vi "Read Connection Information.vi"(8 "error in (no error)":errorcluster, 11 "TwinCAT ADS in":refnum<class "TwinCAT ADS.lvclass">) -> (0 "error out":errorcluster, 1 "Connection Information":T1, 3 "TwinCAT ADS out":refnum<class "TwinCAT ADS.lvclass">)   [LabVIEW 2018, in "TwinCAT ADS.lvclass"]
uses:
  TwinCAT ADS.lvclass
  Controls/Connection Information.ctl
  Controls/Address.ctl
  Controls/Connection Protocol.ctl
  Controls/Router State.ctl
  Controls/Connection State.ctl
  TwinCAT ADS.lvclass/TwinCAT ADS.ctl
  TwinCAT.Ads
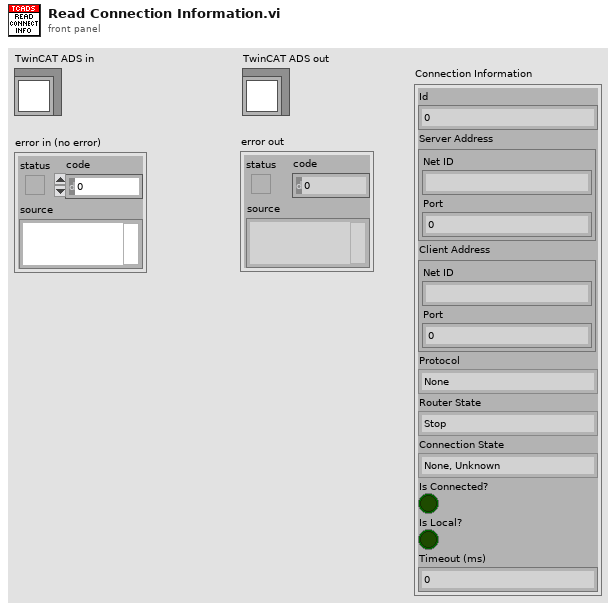
[diagram p1: front panel]
types:
  T1 = typedef "TwinCAT ADS.lvclass/Connection Information.ctl" = cluster{"Id":i32, "Server Address":T2, "Client Address":cluster{"Net ID":string, "Port":i32}, "Protocol":T3, "Router State":T4, "Connection State":T5, "Is Connected?":bool, "Is Local?":bool, "Timeout (ms)":i32}
  T2 = typedef "TwinCAT ADS.lvclass/Address.ctl" = cluster{"Net ID":string, "Port":i32}
  T3 = typedef "TwinCAT ADS.lvclass/Connection Protocol.ctl" = enum16{"None", "Router", "TCP/IP", "All"}
  T4 = typedef "TwinCAT ADS.lvclass/Router State.ctl" = enum16{"Stop", "Start", "Removed", "Unknown"}
  T5 = typedef "TwinCAT ADS.lvclass/Connection State.ctl" = enum16{"None, Unknown", "Disconnected", "Connected", "Lost"}
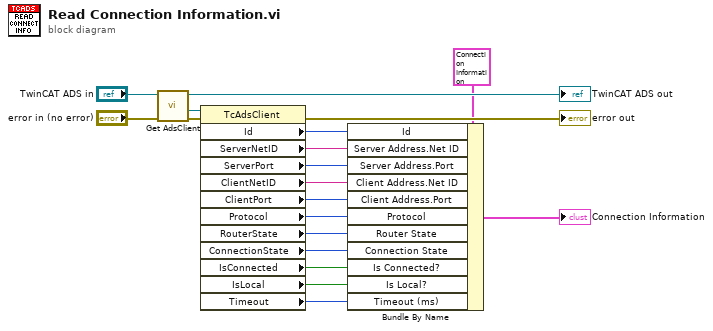
[diagram p0: block diagram]
diagram:
  n1 = call "Get AdsClient.vi"("error in (no error)"="error in (no error)", "TwinCAT ADS in"="TwinCAT ADS in") -> ("error out"=w3:errorcluster, ".NET TcAdsClient"=w2:refnum<k24>, "TwinCAT ADS out"=→"TwinCAT ADS out":refnum<class "TwinCAT ADS.lvclass">)  [unwired: 7 in]
  n2 = property class="TcAdsClient"(reference=w2, error in=w3) -> (error out=→"error out":errorcluster, "Id"=w14:i32, "ServerNetID"=w13:string, "ServerPort"=w12:i32, "ClientNetID"=w11:string, "ClientPort"=w10:i32, "Protocol"=w9:i32, "RouterState"=w8:i32, "ConnectionState"=w4:i32, "IsConnected"=w5:bool, "IsLocal"=w6:bool, "Timeout"=w7:i32)  [unwired: 1 out]
  n3 = Bundle By Name(cluster=T1 {"Id"=0, "Server Address"={"Net ID"="", "Port"=0}, "Client Address"={"Net ID"="", "Port"=0}, "Protocol"=enum."None", "Router State"=enum."Stop", "Connection State"=enum."None, Unknown", "Is Connected?"=FALSE, "Is Local?"=FALSE, "Timeout (ms)"=0} ("Connectio Information"), "Id"=w14, "Server Address.Net ID"=w13, "Server Address.Port"=w12, "Client Address.Net ID"=w11, "Client Address.Port"=w10, "Protocol"=w9, "Router State"=w8, "Connection State"=w4, "Is Connected?"=w5, "Is Local?"=w6, "Timeout (ms)"=w7) -> (→"Connection Information":T1)
